vi "fgv_tim571-tcp.vi"(7 "cmd":T1(ring), 8 "error in":errorcluster, 10 "write data":string, 11 "ip addr":string) -> (0 "error out":errorcluster, 3 "data out":string)   [LabVIEW 2019]
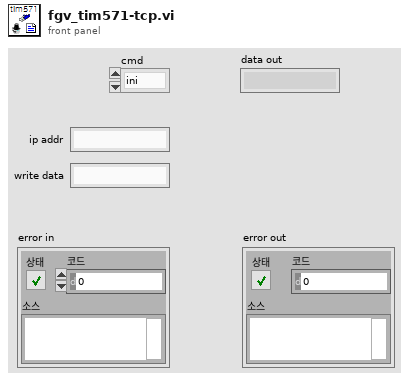
[diagram p1: front panel]
types:
  T1 = enum16{"ini", "write scan-cmd", "write", "read", "close"}
  T2 = enum16{"Standard", "Buffered", "CRLF", "Immediate"}
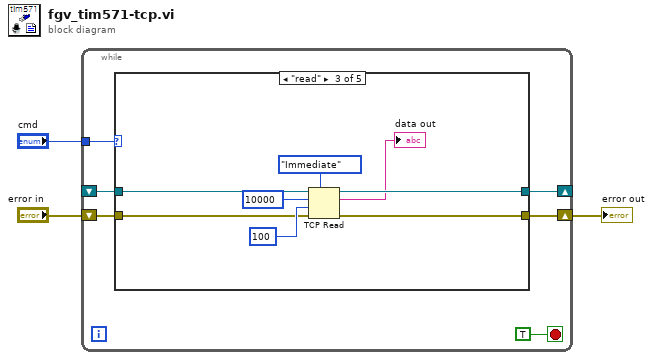
[diagram p0: block diagram]
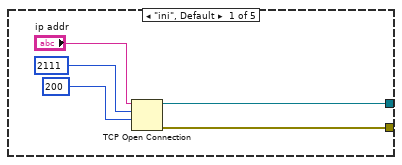
[diagram p2: hidden frame]
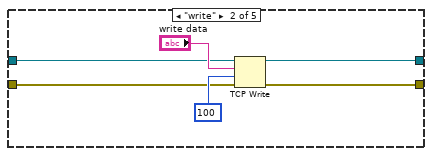
[diagram p3: hidden frame]
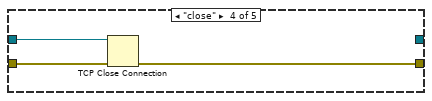
[diagram p4: hidden frame]
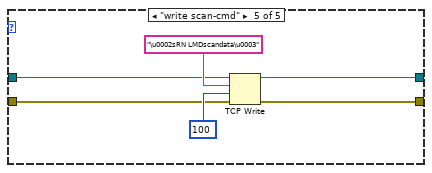
[diagram p5: hidden frame]
diagram:
  n1 = while {
    tunnel: "cmd" -> [w8]
    shift-right: [w5] -> _
    shift-left: _ -> [w6]
    shift-right: [w4] -> w1
    shift-left: "error in" -> [w7]
    stop <- TRUE stop-if-true
    n2 = case shown="\"read\"" w8 {
      tunnel: w7 -> [_ w17 w24 w30 w33]
      tunnel: w6 -> [_ w18 w25 w31 w35]
      tunnel: [w13 w15 w23 _ w34] -> w5
      tunnel: [w10 w16 w22 w29 w32] -> w4
      frame "ini", Default {
        n3 = TCP Open Connection(address="ip addr", remote port or service name=u16 2111 ("원격 포트 또는 서비스 이름"), timeout ms (60000)=200 ("타임아웃 ms (60000)")) -> (connection ID=w13:refnum<k5>, error out=w10:errorcluster)  [unwired: 2 in]
      }
      frame "write" {
        n4 = TCP Write(connection ID=w18, data in="write data", error in (no error)=w17, 9:100 ("타임아웃 ms (25000)")) -> (connection ID out=w15:refnum<k5>, error out=w16:errorcluster)  [unwired: 1 out]
      }
      frame "read" {
        n5 = TCP Read(connection ID=w25, bytes to read=10000, error in (no error)=w24, 7:T2."Immediate" ("mode (standard)"), 9:100 ("타임아웃 ms (25000)")) -> (connection ID out=w23:refnum<k5>, data out=→"data out":string, error out=w22:errorcluster)
      }
      frame "close" {
        n6 = TCP Close Connection(connection ID=w31, error in (no error)=w30) -> (error out=w29:errorcluster)  [unwired: 1 in, 1 out]
      }
      frame "write scan-cmd" {
        n7 = TCP Write(connection ID=w35, data in="\u0002sRN LMDscandata\u0003", error in (no error)=w33, 9:100 ("타임아웃 ms (25000)")) -> (connection ID out=w34:refnum<k5>, error out=w32:errorcluster)  [unwired: 1 out]
      }
    }
  }
  "error out" <- w1
